vi "IEE 754 binary to SGL.vi"(8 "Numeric":i32, 9 "Numeric 2":i32, 10 "Numeric 3":i32, 11 "Numeric 4":i32) -> (2 "Decimal Number":sgl)   [LabVIEW 2015]
panel:
  out "x << y 6":u32 format="%.0b"
  out "x << y 5":u32 format="%.0b"
  out "x << y 3":u32 format="%.0b"
  out "x << y 2":u32 format="%11b"
  out "x << y":u32 format="%.0b"
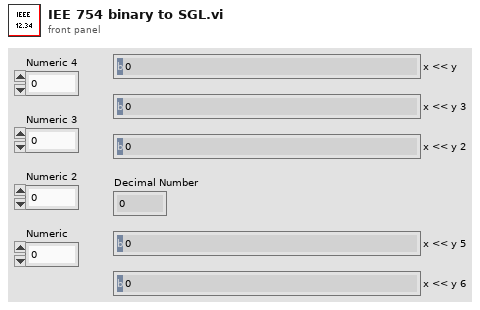
[diagram p1: front panel]
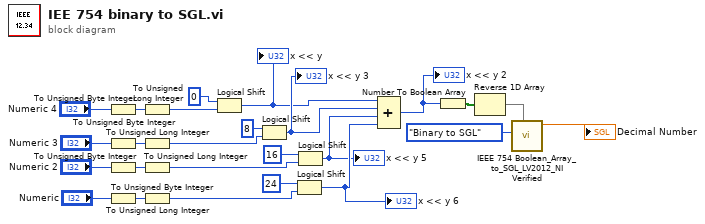
[diagram p0: block diagram]
diagram:
  n1 = To Unsigned Byte Integer(number="Numeric 4") -> (unsigned 8bit integer=w1:u8)
  n2 = To Unsigned Byte Integer(number="Numeric 3") -> (unsigned 8bit integer=w2:u8)
  n3 = To Unsigned Byte Integer(number="Numeric 2") -> (unsigned 8bit integer=w3:u8)
  n4 = To Unsigned Byte Integer(number="Numeric") -> (unsigned 8bit integer=w4:u8)
  n5 = To Unsigned Long Integer(number=w1) -> (unsigned 32bit integer=w5:u32)
  n6 = To Unsigned Long Integer(number=w2) -> (unsigned 32bit integer=w9:u32)
  n7 = To Unsigned Long Integer(number=w3) -> (unsigned 32bit integer=w10:u32)
  n8 = To Unsigned Long Integer(number=w4) -> (unsigned 32bit integer=w15:u32)
  n9 = Logical Shift(y=i16 0, x=w5) -> (x << y=w11:u32)
  "x << y" <- w11
  n10 = Logical Shift(y=i16 8, x=w9) -> (x << y=w12:u32)
  "x << y 3" <- w12
  n11 = Logical Shift(y=i16 24, x=w15) -> (x << y=w16:u32)
  "x << y 6" <- w16
  n12 = Logical Shift(y=i16 16, x=w10) -> (x << y=w13:u32)
  "x << y 5" <- w13
  n13 = Compound Arithmetic op=ADD(w11, w12, w13, w16) -> (w18:u32)
  "x << y 2" <- w18
  n14 = Number To Boolean Array(number=w18) -> (Boolean array=w21:bool[])
  n15 = Reverse 1D Array(array=w21) -> (reversed array=w19:bool[])
  n16 = call "IEEE 754 Boolean_Array_to_SGL_LV2012_NI Verified.vi"("array bool"=w19, "Tab Control"=enum32{"SGL to Binary", "Binary to SGL"}."Binary to SGL") -> ("Decimal Number"=→"Decimal Number":sgl)  [unwired: 9 in]
